vi "Generate Rectangle Sequence Images.vi"(6 "Predominant ROI type":T1=enum."Comp. volume", 7 "Imaging Protocol":T2=enum."Live Imaging", 8 "error in (no error)":errorcluster, 9 "Use connector pane path input":bool, 11 "TDMS file path & name":path) -> (0 "error out":errorcluster, 2 "Destination fiolder":path, 3 "tdms file to close":refnum<k34>)   [LabVIEW 2013]
uses:
  Typedefs/Imaging Protocols enum.ctl
  Typedefs/ROI ID Enum.ctl
  User Interface/Visualisation/Functional Imaging Viewer/SubVIs/Experiment header interface/Typedefs/Save-Load-Save as-Load last enum.ctl
  User Interface/Visualisation/Functional Imaging Viewer/SubVIs/Experiment header interface/Typedefs/Header file type enum.ctl
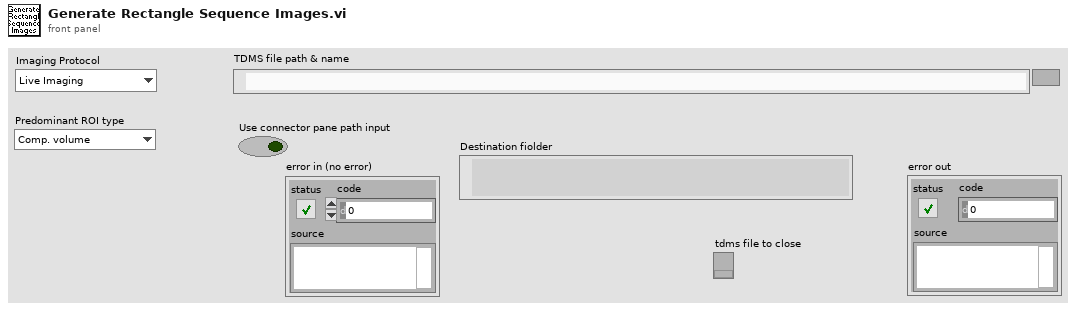
[diagram p1: front panel]
types:
  T1 = typedef "ROI ID Enum.ctl" = enum16{"Point", "MiniScan", "Comp. MiniScan", "Rectangle", "Comp. volume", "Arb. plane point"}
  T2 = typedef "Imaging Protocols enum.ctl" = enum16{"AOL Z-Stack", "Motor Z Stack", "Functional Acquisition", "Single Plane Acquisition", "Volume Acquisition", "Live Imaging", "Live Plane Imaging", "Live Volume Imaging"}
  T3 = typedef "Header file type enum.ctl" = enum16{"All parameters", "Params for funct acq w ROI or mscn", "Params for funct acq w rectangles", "Live imaging header parameters", "AOL Parameters"}
  T4 = typedef "Save-Load-Save as-Load last enum.ctl" = enum16{"Save file", "Save file as", "Load file", "Load last file"}
  T5 = typedef "Header parameters cluster-ALL.ctl" = cluster{"Imaging Protocol":T2, "Number of POI":u16, "Number of Miniscans":u16, "Number of Trials":u16, "Number of Cycles ":u64, "# Averaged Frames":u16, "Laser power (%)":u8, "Pockels":dbl, "Acquisition Length (sec)":dbl, "Fill time (us)":dbl, "POI Dwell time (us)":dbl, "Miniscan Dwell time per pixel (us)":dbl, "PMT 1":dbl, "PMT 2":dbl, "Back Apperture":dbl, "Zoom":dbl, "Frame Size":T6, "Center Frequency":dbl, "Field of View":dbl, "DwellTime (us)":dbl, "Wavelength (nm)":dbl, "AOL Z":dbl, "AOL Mode":T7, "GridXY":dbl, "GridZ":dbl, "TriggerDelay (sec)":dbl, "Number of Pixels in Miniscan":u16, "Experiment folder path":path, "X centre":dbl, "Y centre":dbl, "Angle (degrees)":dbl, "Plane Mode":T8, "Software version":dbl, "Objective":T9, "MotorZ Calibration":u32, "Pockels Calibration":u32, "Threshold":u16[], "Video length (sec)":dbl, "Frame rate (fps)":u8, "Rectangle ROI length (pixels)":u16, "Rectangle ROI height (pixels)":u16}
  T6 = typedef "Frame Size.ctl" = u16
  T7 = typedef "AOL modes.ctl" = enum16{"Raster", "Structural", "Pointing", "Mini Scan", "Alignment"}
  T8 = typedef "Plane Mode.ctl" = u16
  T9 = typedef "Objective selector control enum.ctl" = string
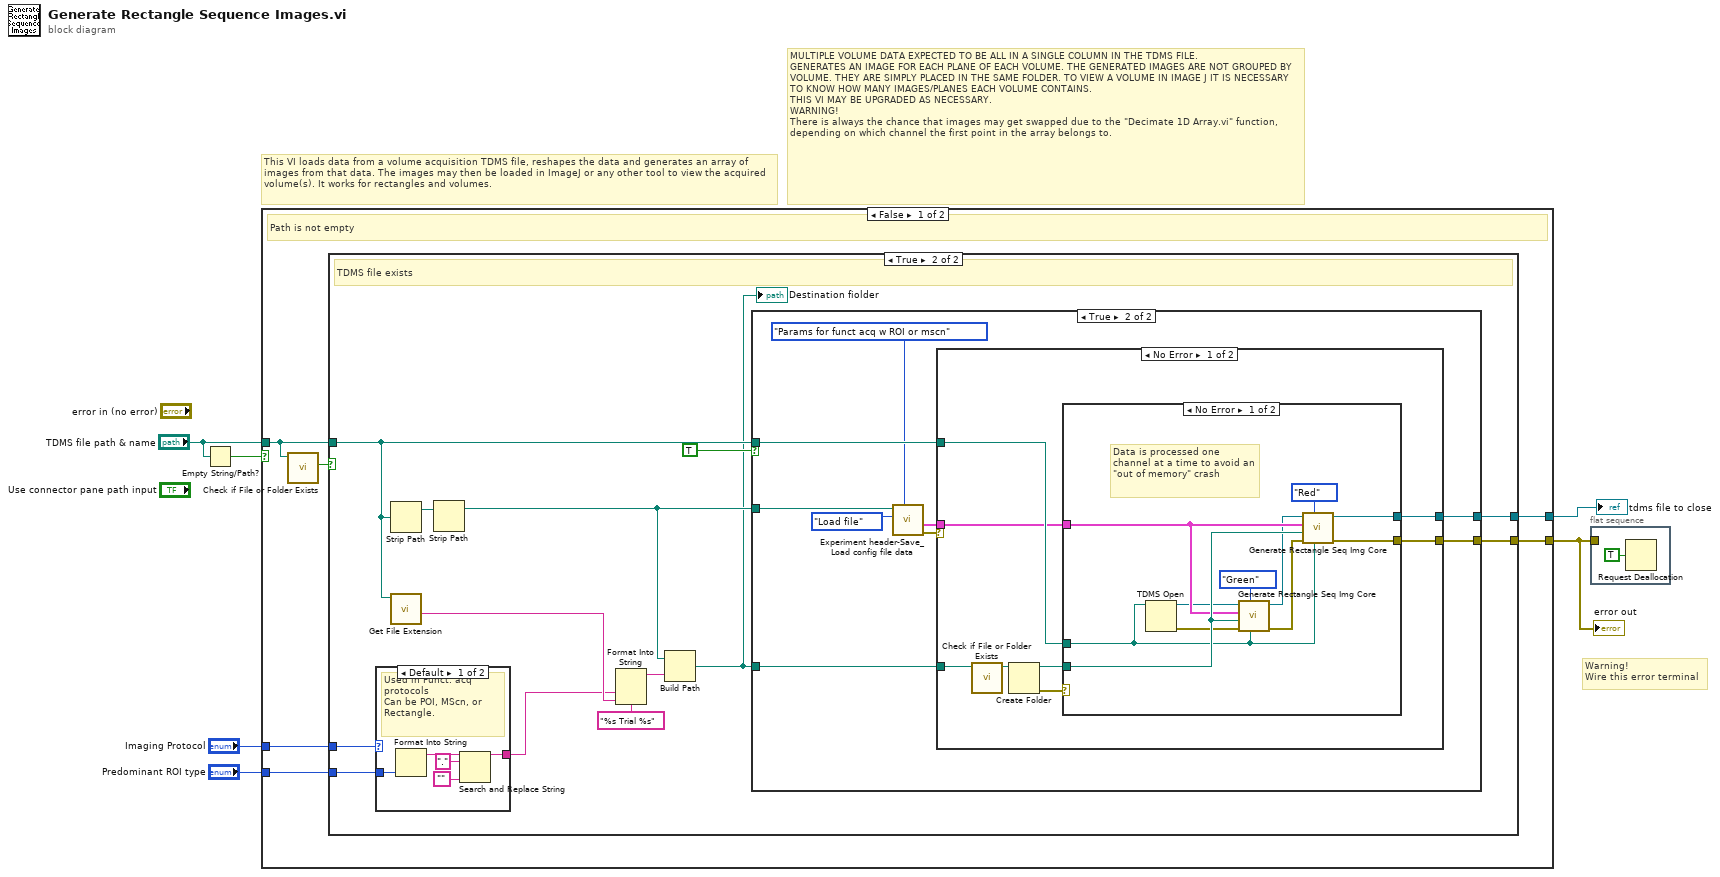
[diagram p0: block diagram]
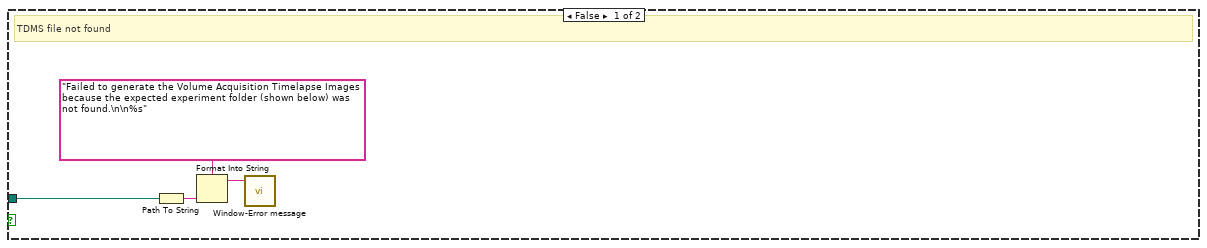
[diagram p2: hidden frame]
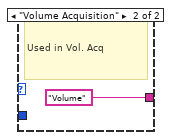
[diagram p3: hidden frame]
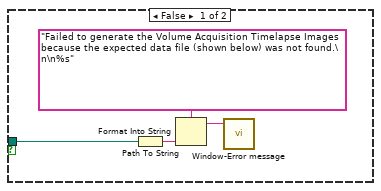
[diagram p4: hidden frame]
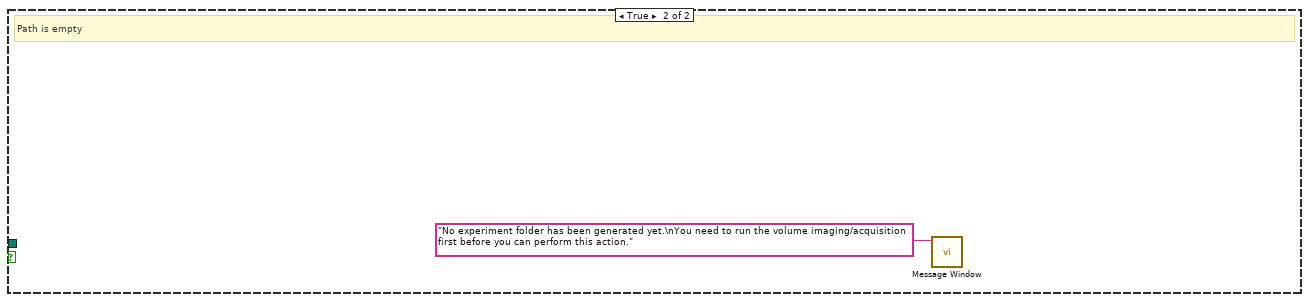
[diagram p7: hidden frame]
diagram:
  # "This VI loads data from a volume acquisition TDMS file, reshapes the data and generates an array of images from that data. The images may then be loaded in ImageJ or any other tool to view the acquired volume(s). It works for rectangles and volumes."
  # "Warning!\nWire this error terminal"
  # "MULTIPLE VOLUME DATA EXPECTED TO BE ALL IN A SINGLE COLUMN IN THE TDMS FILE.\nGENERATES AN IMAGE FOR EACH PLANE OF EACH VOLUME. THE GENERATED IMAGES ARE NOT GROUPED BY VOLUME. THEY ARE SIMPLY PLACED IN THE SAME FOLDER. TO VIEW A VOLUME IN IMAGE J IT IS NECESSARY TO KNOW HOW MANY IMAGES/PLANES EACH VOLUME CONTAINS.\nTHIS VI MAY BE UPGRADED AS NECESSARY.\nWARNING!\nThere is always the chance that images may get swapped due to the \"Decimate 1D Array.vi\" function, depending on which channel the first point in the array belongs to."
  n1 = Empty String/Path?(string/path="TDMS file path & name") -> (empty?=w6:bool)
  n2 = case shown="False" w6 {
    tunnel: "TDMS file path & name" -> [w11 _]
    tunnel: [w10 _] -> w2
    tunnel: "Imaging Protocol" -> [w9 _]
    tunnel: "Predominant ROI type" -> [w8 _]
    tunnel: [w7 _] -> w1
    frame False {
      # "Path is not empty"
      n3 = call <vilib>:"Check if File or Folder Exists.vi"("path"=w11) -> ("file or folder exists?"=w12:bool)  [unwired: 8 in, 2 out]
      n4 = case shown="True" w12 {
        tunnel: w11 -> [w15 w28]
        tunnel: [_ w26] -> w10
        tunnel: w9 -> [_ w24]
        tunnel: w8 -> [_ w23]
        tunnel: [_ w22] -> w7
        frame False {
          # "TDMS file not found"
          n5 = Path To String(path=w15) -> (string=w14:string)
          n6 = Format Into String(format string="Failed to generate the Volume Acquisition Timelapse Images because the expected experiment folder (shown below) was not found.\n\n%s", w14) -> (resulting string=w13:string)  [unwired: 2 in, 1 out]
          n7 = call "Window-Error message.vi"("Message"=w13) -> ()  [unwired: 10 in, 1 out]
        }
        frame True {
          # "TDMS file exists"
          n8 = case shown="Default" w24 {
            tunnel: w23 -> [w34 _]
            tunnel: [w30 "Volume" ("result string")] -> w18
            frame Default {
              # "Used in Funct. acq protocols\nCan be POI, MScn, or Rectangle."
              n9 = Format Into String(w34) -> (resulting string=w33:string)  [unwired: 3 in, 1 out]
              n10 = Search and Replace String(input string=w33, search string=".", replace string="" ("replace string (\"\")")) -> (result string=w30:string)  [unwired: 5 in, 3 out]
            }
            frame "Volume Acquisition" {
              # "Used in Vol. Acq"
            }
          }
          n11 = Strip Path(path=w28) -> (stripped path=w21:path)  [unwired: 1 out]
          n12 = call <vilib>:"Get File Extension.vi"("file"=w28) -> ("filename without extension"=w19:string)  [unwired: 7 in, 3 out]
          n13 = Strip Path(path=w21) -> (stripped path=w27:path)  [unwired: 1 out]
          n14 = Format Into String(format string="%s Trial %s", w18, w19) -> (resulting string=w17:string)  [unwired: 2 in, 1 out]
          n15 = Build Path(base path=w27, name or relative path=w17) -> (appended path=w25:path)
          "Destination fiolder" <- w25
          n16 = case shown="True" TRUE ("file or folder exists?") {
            tunnel: w25 -> [_ w48]
            tunnel: w27 -> [_ w44]
            tunnel: w28 -> [w36 w47]
            tunnel: [_ w41] -> w26
            tunnel: [_ w40] -> w22
            frame False {
              n17 = Path To String(path=w36) -> (string=w37:string)
              n18 = Format Into String(format string="Failed to generate the Volume Acquisition Timelapse Images because the expected data file (shown below) was not found.\n\n%s", w37) -> (resulting string=w38:string)  [unwired: 2 in, 1 out]
              n19 = call "Window-Error message.vi"("Message"=w38) -> ()  [unwired: 10 in, 1 out]
            }
            frame True {
              n20 = call "Experiment header-Save_Load config file data.vi"("Header file type"=Header_file_type_enum."Params for funct acq w ROI or mscn", "Function"=Save-Load-Save_as-Load_last_enum."Load file", "Experiment data folder path"=w44) -> ("error out"=w43:errorcluster, "All header parameters out"=w45:T5)  [unwired: 7 in]
              n21 = case shown="No Error" w43 {
                tunnel: w48 -> [w56 _]
                tunnel: w47 -> [w55 _]
                tunnel: w45 -> [w51 _]
                tunnel: [w52 _] -> w41
                tunnel: [w50 _] -> w40
                frame No Error {
                  n22 = call <vilib>:"Check if File or Folder Exists.vi"("path"=w56) -> ("dup path"=w49:path)  [unwired: 8 in, 2 out]
                  n23 = Create Folder(path (use dialog)=w49) -> (created path=w53:path, error out=w54:errorcluster)  [unwired: 2 in, 1 out]
                  n24 = case shown="No Error" w54 {
                    selector: w54 -> [_ w68]
                    tunnel: w53 -> [w67 _]
                    tunnel: w55 -> [w59 _]
                    tunnel: w51 -> [w66 _]
                    tunnel: [w58 w68] -> w52
                    tunnel: [w57 _] -> w50
                    frame No Error {
                      # "Data is processed one channel at a time to avoid an \"out of memory\" crash"
                      n25 = TDMS Open(11:w59) -> (0:w61:errorcluster, 3:w60:refnum<k34>)  [unwired: 6 in]
                      n26 = call "Generate Rectangle Seq Img Core.vi"("TDMS file path & name"=w59, "Channel to process"=enum16{"Red", "Green"}."Green", "error in (no error)"=w61, "<Vol images/video folder>"=w67, "All header parameters"=w66, "tdms file ref"=w60) -> ("error out"=w65:errorcluster, "tdms file out"=w62:refnum<k34>)  [unwired: 4 in]
                      n27 = call "Generate Rectangle Seq Img Core.vi"("TDMS file path & name"=w59, "Channel to process"=enum16{"Red", "Green"}."Red", "error in (no error)"=w65, "<Vol images/video folder>"=w67, "All header parameters"=w66, "tdms file ref"=w62) -> ("error out"=w58:errorcluster, "tdms file out"=w57:refnum<k34>)  [unwired: 4 in]
                    }
                    frame Error {
                    }
                  }
                }
                frame Error {
                  # "Error reporting handled inside the subVI."
                }
              }
            }
          }
        }
      }
    }
    frame True {
      # "Path is empty"
      n28 = call "Message Window.vi"("Message string"="No experiment folder has been generated yet.\nYou need to run the volume imaging/acquisition first before you can perform this action.") -> ()  [unwired: 10 in, 1 out]
    }
  }
  "error out" <- w2
  "tdms file to close" <- w1
  n29 = flat-sequence {
    tunnel: w2 -> [_]
    frame #0 {
      n30 = Request Deallocation(TRUE ("flag")) -> ()
    }
  }
